vi "BeadCoolerFixedZ(SubVI)_noint_extraHP.vi"(1 "AI0":i16, 2 "Dc Pos":i16, 7 "dg":fxp<+/-,24,12>, 8 "hp coeff":i32[](array[numeric])=[946630756, 1010186290], 12 "lp coeff":i32[](array[numeric])=[1008310688, 32715568], 13 "Upper lim":fxp<+/-,16,16>, 14 "Lower lim":fxp<+/-,16,16>) -> (10 "Output":fxp<+/-,16,16>)   [LabVIEW 2016]
uses:
  <vilib>/rvi/FXPMathLib/FxpInterpret/XNode/nifxpmath_Interpret.xnode
  <vilib>/rvi/Analysis/measure/butterworth/XNode/niFpgaButterworthFilter.xnode
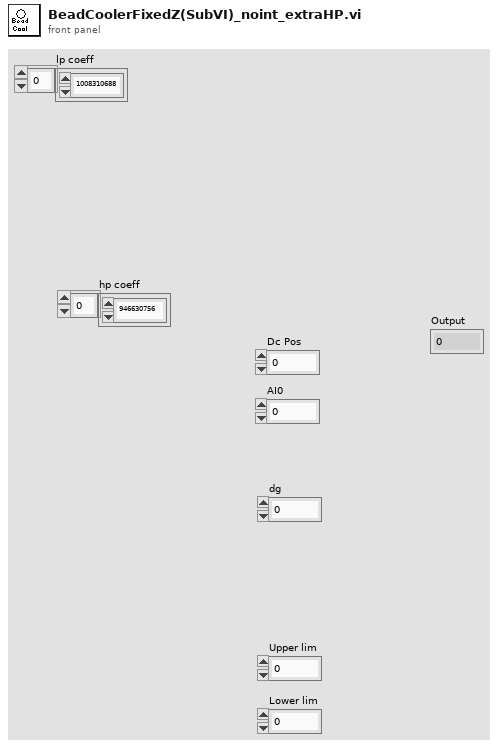
[diagram p1: front panel]
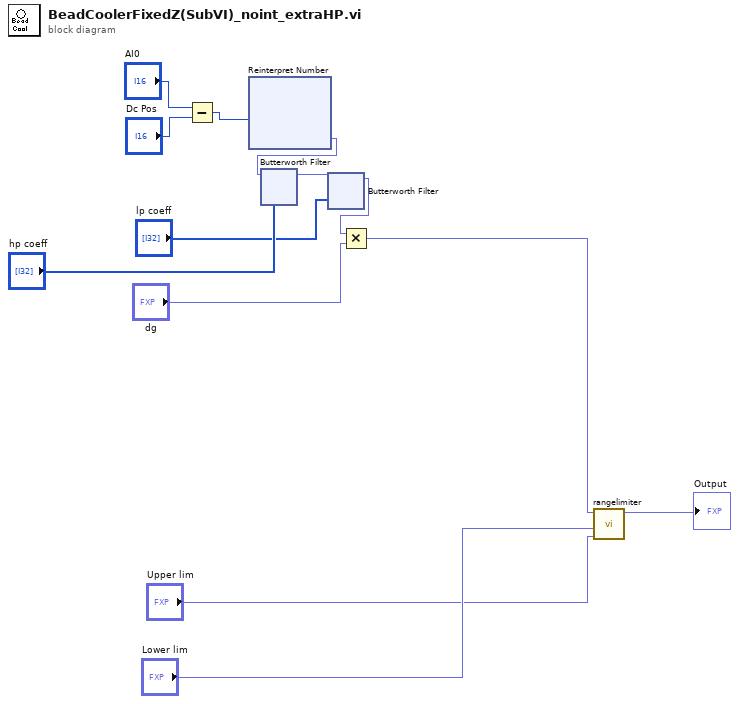
[diagram p0: block diagram]
diagram:
  n1 = Subtract(x="AI0", y="Dc Pos") -> (x-y=w9:i16)
  n2 = xnode "Reinterpret Number"("x"=w9) -> ("y"=w1:fxp<+/-,16,16>)
  n3 = xnode "Butterworth Filter"("input data"=w1, "scaled coefficients"="hp coeff") -> ("output data"=w5:fxp<+/-,16,16>)  [unwired: 1 in]
  n4 = xnode "Butterworth Filter"("input data"=w5, "scaled coefficients"="lp coeff") -> ("output data"=w4:fxp<+/-,16,16>)  [unwired: 1 in]
  n5 = Multiply(x=w4, y="dg") -> (x*y=w2:fxp<+/-,16,16>)
  n6 = call "rangelimiter.vi"("Upper lim"="Upper lim", "Lower lim"="Lower lim", "Input"=w2) -> ("Output"=→"Output":fxp<+/-,16,16>)  [unwired: 8 in]
